vi "PKG_IMC_FindNetCard.vi"(10 "num":i32, 11 "info":string) -> (1 "function return":i32, 2 "num out":i32, 3 "info out":string)   [LabVIEW 2011, in "IMC_Pkg4xxx.lvlib"]
doc: "PKG_IMC_FindNetCard (char info[16][256], int* num) ;"
uses:
  IMC_Pkg4xxx.lvlib
  IMC_Pkg4xxx.dll
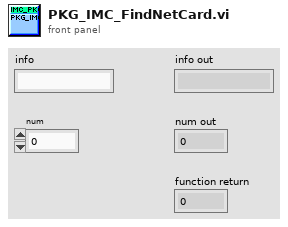
[diagram p1: front panel]
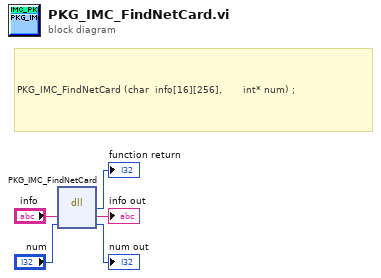
[diagram p0: block diagram]
diagram:
  # "PKG_IMC_FindNetCard (char  info[16][256],\t\t\t\t\t\t\tint* num) ;"
  n1 = dll-call lib="PTH1mabs F光盘刻录\niMC MotionIMCNet_V4.0IMCAppincLabviewIMC_PKG4xxxIMC_PKG4xxx\nIMC_Pkg4xxx.*" fn="PKG_IMC_FindNetCard"("info"="info", "num"="num") -> (→"function return":i32, "info"=→"info out":string, "num"=→"num out":i32)  [unwired: 3 in, 2 out]
